vi "Insert_Reposition Node Vertically.vi"(8 "error in":errorcluster, 9 "Node in":refnum<vi>, 11 "Vertical Change":i32) -> (0 "error out":errorcluster, 1 "Node out":refnum<vi>)   [LabVIEW 2020]
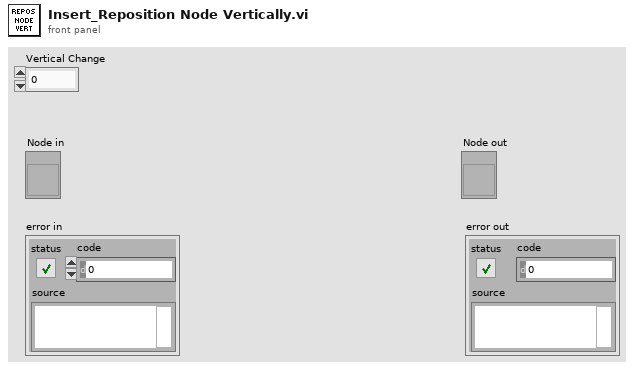
[diagram p1: front panel]
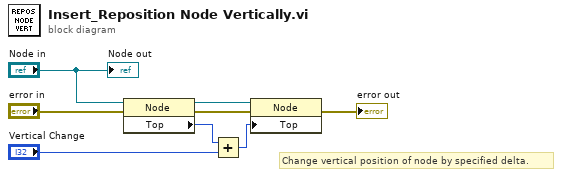
[diagram p0: block diagram]
diagram:
  # "Change vertical position of node by specified delta."
  n1 = property class="Node"(reference="Node in", error in="error in") -> (reference out=w3:refnum<vi>, error out=w2:errorcluster, "Top"=w4:i32)
  n2 = Add(x=w4, y="Vertical Change") -> (x+y=w5:i32)
  n3 = property class="Node"(reference=w3, error in=w2, "Top"=w5) -> (error out=→"error out":errorcluster)  [unwired: 1 out]
  "Node out" <- "Node in"
